vi "ToggleTab.vi"(8 "Error In":errorcluster, 10 "Tab Index":i32, 11 "TabCtl Refnum":refnum<vi>) -> (0 "Error Out":errorcluster)   [LabVIEW 2017, in "Client.lvlib" / "UI_API.lvlib"]
uses:
  UI_API.lvlib
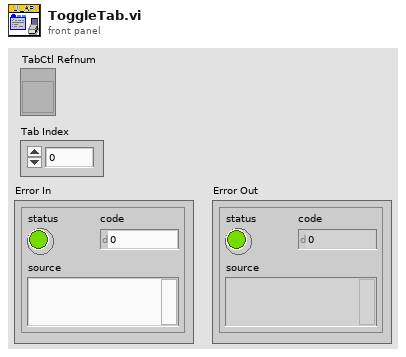
[diagram p1: front panel]
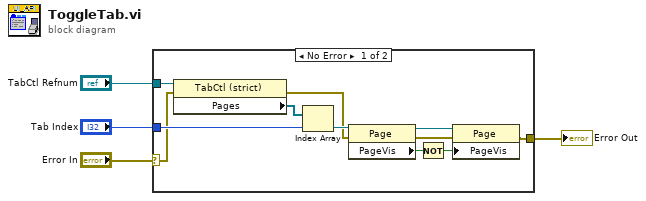
[diagram p0: block diagram]
diagram:
  n1 = case shown="No Error" "Error In" {
    selector: "Error In" -> [w11 w16]
    tunnel: "Tab Index" -> [w15 _]
    tunnel: [w5 w16] -> w2
    tunnel: "TabCtl Refnum" -> [w14 _]
    frame No Error {
      n2 = property class="TabCtl (strict)"(reference=w14, error in=w11) -> (error out=w7:errorcluster, "Pages"=w13:refnum<vi>[])  [unwired: 1 out]
      n3 = Index Array(array=w13, index=w15) -> (element=w12:refnum<vi>)
      n4 = property class="Page"(reference=w12, error in=w7) -> (reference out=w10:refnum<vi>, error out=w6:errorcluster, "PageVis"=w9:bool)
      n5 = Not(x=w9) -> (.not. x?=w8:bool)
      n6 = property class="Page"(reference=w10, error in=w6, "PageVis"=w8) -> (error out=w5:errorcluster)  [unwired: 1 out]
    }
    frame Error {
    }
  }
  "Error Out" <- w2
